vi "Set Bounds.vi"(8 "error in (no error)":errorcluster, 10 "Bounds":T1, 11 "GUI Helper in":refnum<class "MessageQ.lvclass">) -> (0 "error out":errorcluster, 3 "GUI Helper out":refnum<class "MessageQ.lvclass">)   [LabVIEW 2020, in "VolatusGUI.lvlib" / "GUI Helper.lvclass"]
uses:
  GUI Helper.lvclass
  Volatus/MessageQ/MessageQ.lvclass
  <vilib>/Utility/miscctls.llb/LVRectTypeDef.ctl
  Bounds Message.ctl
  Volatus/MessageQ/MessageQ.lvclass/MessageQ.ctl
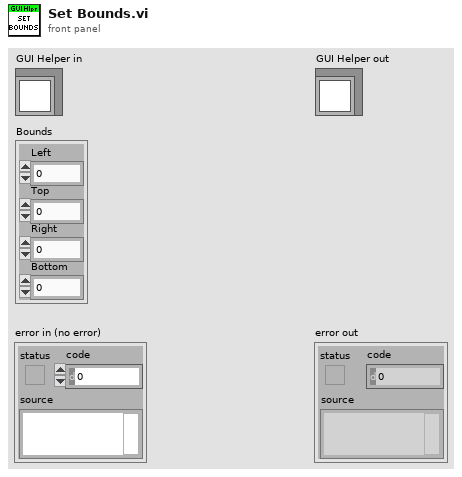
[diagram p1: front panel]
types:
  T1 = typedef "LVRectTypeDef.ctl" = cluster{"Left":i16, "Top":i16, "Right":i16, "Bottom":i16}
  T2 = typedef "VolatusGUI.lvlib/GUI Helper.lvclass/Bounds Message.ctl" = cluster{"Bounds":T1}
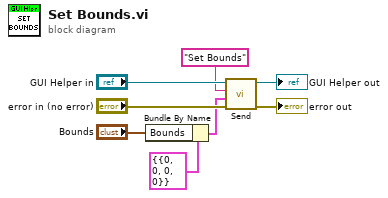
[diagram p0: block diagram]
diagram:
  n1 = Bundle By Name(cluster=T2 {"Bounds"={"Left"=0, "Top"=0, "Right"=0, "Bottom"=0}} ("Bound Message"), "Bounds"="Bounds") -> (w1:T2)
  n2 = call "Send.vi"("error in (no error)"="error in (no error)", "Data"=w1, "ID"="Set Bounds", "MessageQ in"="GUI Helper in") -> ("error out"=→"error out":errorcluster, "MessageQ out"=→"GUI Helper out":refnum<class "MessageQ.lvclass">)  [unwired: 6 in]
